vi "RemoveStartupTrendPoints.vi"(8 "error in (no error)":errorcluster, 9 "Group":T1, 11 "TrendPoints in":T5[](array[typedef])) -> (0 "error out":errorcluster, 3 "TrendPoints out":T5[](array[typedef]))   [LabVIEW 2017, in "McsaStartupAnalysis.lvlib"]
uses:
  <vilib>/addons/InsightCM/Devices/Shared/Mcsa/McsaStartupAnalysis/McsaStartupAnalysis.lvlib
  <vilib>/addons/InsightCM/MessageBus/Base/controls/TrendPoint.ctl
  <vilib>/addons/InsightCM/MessageBus/Base/controls/KeyValuePair.ctl
  <vilib>/addons/InsightCM/Devices/Shared/Mcsa/McsaStartupAnalysis/controls/Group.ctl
  <vilib>/addons/InsightCM/Devices/Shared/Mcsa/McsaStartupAnalysis/controls/ChannelForStartup.ctl
  <vilib>/addons/InsightCM/Devices/Shared/Mcsa/McsaStartupAnalysis/controls/StartupFeature.ctl
  <vilib>/addons/InsightCM/Devices/Shared/Mcsa/McsaStartupAnalysis/controls/MotorInfo.ctl
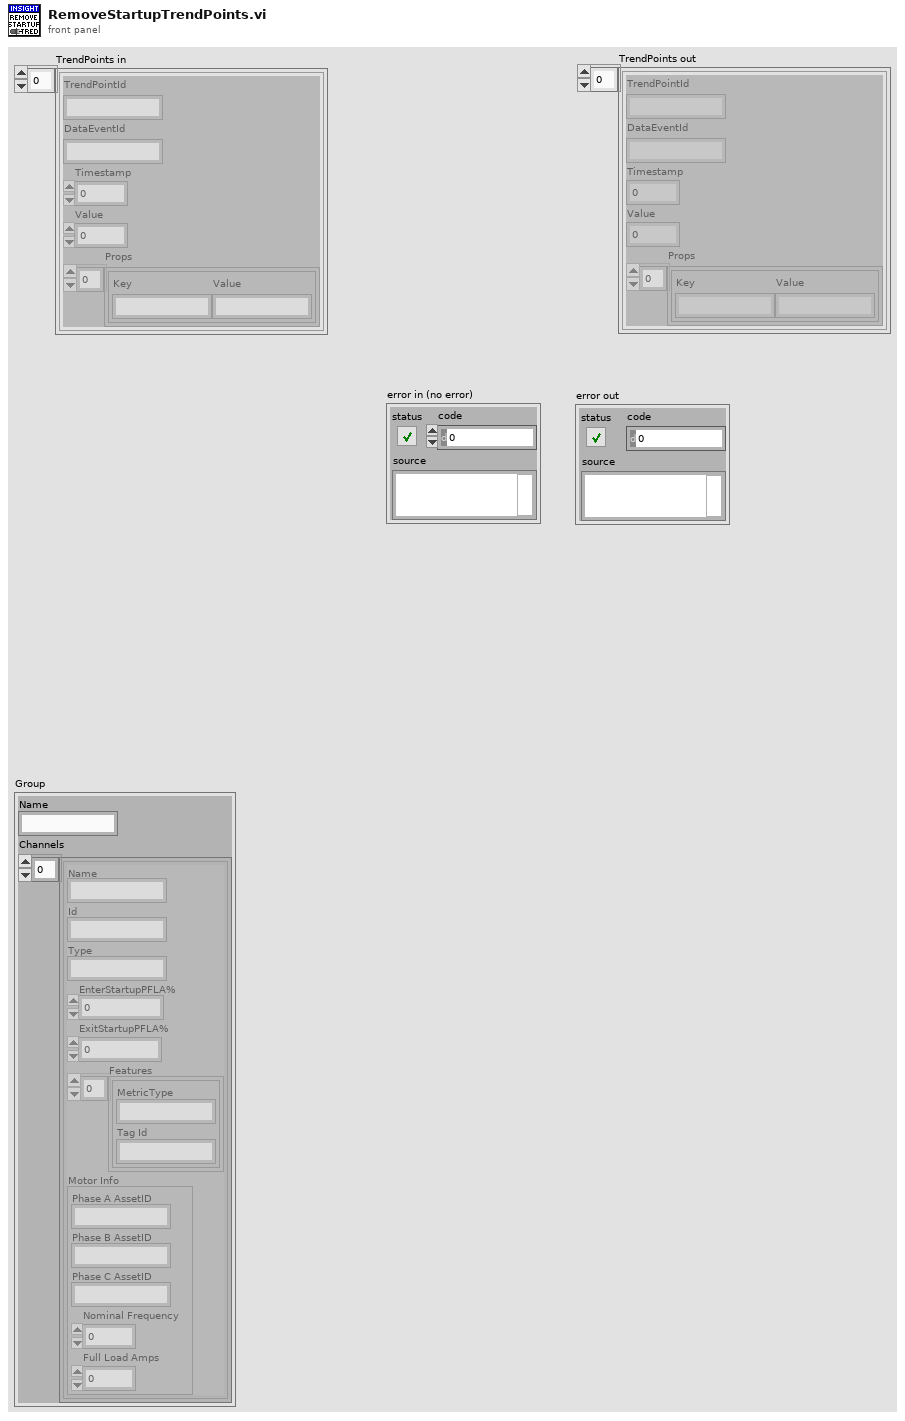
[diagram p1: front panel]
types:
  T1 = typedef "McsaStartupAnalysis.lvlib/Group.ctl" = cluster{"Name":string, "Channels":T2[]}
  T2 = typedef "McsaStartupAnalysis.lvlib/ChannelForStartup.ctl" = cluster{"Name":string, "Id":string, "Type":string, "EnterStartupPFLA%":dbl, "ExitStartupPFLA%":dbl, "Features":T3[], "Motor Info":T4}
  T3 = typedef "McsaStartupAnalysis.lvlib/StartupFeature.ctl" = cluster{"MetricType":string, "Tag Id":string}
  T4 = typedef "McsaStartupAnalysis.lvlib/MotorInfo.ctl" = cluster{"Phase A AssetID":string, "Phase B AssetID":string, "Phase C AssetID":string, "Nominal Frequency":dbl, "Full Load Amps":dbl}
  T5 = typedef "TrendPoint.ctl" = cluster{"TrendPointId":string, "DataEventId":string, "Timestamp":i64, "Value":dbl, "Props":T6[]}
  T6 = typedef "KeyValuePair.ctl" = cluster{"Key":string, "Value":string}
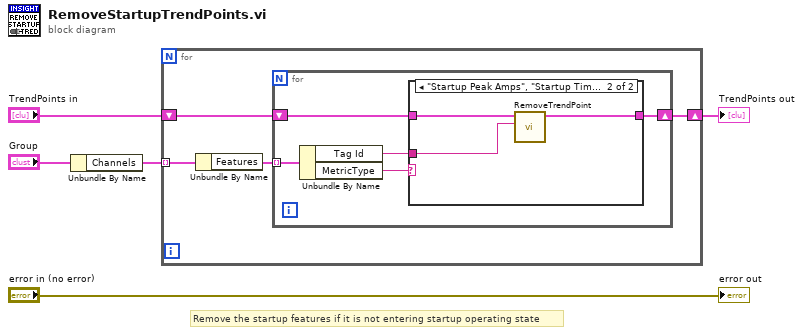
[diagram p0: block diagram]
diagram:
  # "Remove the startup features if it is not entering startup operating state"
  n1 = Unbundle By Name("Group") -> ("Channels"=w3:T2[])
  n2 = for {
    tunnel: w3 -> [w7] mode=indexing
    shift-right: [w8] -> w5
    shift-left: "TrendPoints in" -> [w9]
    n3 = Unbundle By Name(w7) -> ("Features"=w6:T3[])
    n4 = for {
      tunnel: w6 -> [w14] mode=indexing
      shift-right: [w12] -> w8
      shift-left: w9 -> [w13]
      n5 = Unbundle By Name(w14) -> ("Tag Id"=w11:string, "MetricType"=w10:string)
      n6 = case shown="\"Startup Peak Amps\", \"Startup Time\"" w10 {
        tunnel: w13 -> [w15 w18]
        tunnel: [w15 w17] -> w12
        tunnel: w11 -> [_ w16]
        frame Default {
        }
        frame "Startup Peak Amps", "Startup Time" {
          n7 = call <vilib>:"RemoveTrendPoint.vi"("TrendPoints id"=w16, "TrendPoints in"=w18) -> ("TrendPoints out"=w17:T5[])  [unwired: 9 in]
        }
      }
    }
  }
  "TrendPoints out" <- w5
  "error out" <- "error in (no error)"
